vi "DFD FXP NStage MRate Code Generator.vi"(5 "open project? (F)":bool, 6 "confirm? (T)":bool=TRUE, 7 "# channels":i32=1, 8 "error in (no error)":errorcluster, 9 "filter name":string, 10 "destination folder":path, 11 "multirate filters":T1[](array[typedef]) {"mMRate_SumWl" min=1 max=32 step=1; "mMRate_InputIwl" min=1 max=32 step=1; "mMRate_GainWl" min=1 max=32 step=1; "mMRate_OutputWl" min=1 max=32 step=1; "mMRate_InputWl" min=1 max=32 step=1; "mMRate_CoefWl" min=1 max=32 step=1; "mMRate_Mode" items=["Default"=-1, "No Rate Change"=0, "Interpolation"=1, "Decimation"=2, "Interpolated"=3, "Rational"=4]}) -> (0 "error out":errorcluster, 1 "sampling frequency/FPGA clock":dbl, 2 "lvproj path":path)   [LabVIEW 2017, in "NI_DigFilterLicensed.lvlib"]
doc: "Generates LabVIEW field-programmable gate array (FPGA) code from a multistage multirate filter."
uses:
  <vilib>/addons/Digital Filter Design/NI_DigFilterLicensed.lvlib
  <vilib>/addons/Digital Filter Design/_Objects.llb/DFD Multirate Filter Obj.ctl
  <vilib>/addons/Digital Filter Design/_Objects.llb/DFD Multirate Mode.ctl
  <vilib>/addons/Digital Filter Design/_Objects.llb/DFD Coef Norm Type.ctl
  <vilib>/addons/Digital Filter Design/_Objects.llb/DFD Round-off Mode.ctl
  <vilib>/addons/Digital Filter Design/_Objects.llb/DFD FXP MRate Multiply Mode.ctl
  <vilib>/addons/Digital Filter Design/nMAC.llb/Typedefs/dfd_nMAC_Parameter.ctl
  <vilib>/addons/Digital Filter Design/nMAC.llb/Typedefs/dfd_nMAC_Memory Type.ctl
  <vilib>/addons/Digital Filter Design/nMAC.llb/Typedefs/dfd_nMAC_Coef Reload API.ctl
  <vilib>/addons/Digital Filter Design/nMAC.llb/Typedefs/dfd_nMAC_Execution Mode.ctl
  <vilib>/addons/Digital Filter Design/NI_DigFilter_CodeGen.lvlib
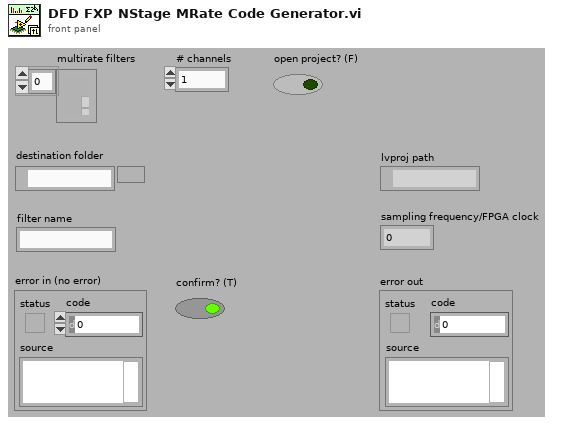
[diagram p1: front panel]
types:
  T1 = typedef "NI_DigFilterLicensed.lvlib/DFD Multirate Filter Obj.ctl" = cluster{"mMRate_Structure":enum16{"CIC", "FIR", "IIR", "Lattice"}, "mMRate_Mode":T2, "mMRate_Factor":i32, "mMRate_FIRParams":cluster{"mMRate_FIR_H":dbl[], "mMRate_FIR_IsNyquist?":bool, "mMRate_FIR_IsSymmetric?":bool}, "mMRate_CICParams":cluster{"mMRate_CIC_#Stage":i32, "mMRate_CIC_Lag":i32, "mMRate_CIC_Type":enum16{"Lowpass", "Highpass"}}, "mMRate_Order":i32, "mMRate_Version":string, "mMRate_Comments":string, "mMRate_RationalFactor":cluster{"mMRate_L":i32, "mMRate_M":i32}, "mMRate_Fs":dbl, "mMRate_Quantized?":bool, "mMRate_QFilterGain":dbl, "mMRate_CoefWl":i16, "mMRate_Scaling":cluster{"mMRate_ScaleByPowerOf2?":bool, "mMRate_ScaleType":T3}, "mMRate_InputWl":i16, "mMRate_OutputWl":i16, "mMRate_OutputMode":T4, "mMRate_MultMode":T5, "mMRate_BitPruning":bool, "mMRate_GainWl":i16, "mMRate_OutputFwl":i16, "mMRate_SumIwl":i16, "mMRate_InputIwl ":i16, "mMRate_SumWl":i16, "mMRate_CoefIwl":i16}
  T2 = typedef "NI_DigFilterLicensed.lvlib/DFD Multirate Mode.ctl" = i16
  T3 = typedef "NI_DigFilterLicensed.lvlib/DFD Coef Norm Type.ctl" = enum16{"No Norm", "Time Domain 1-Norm", "Time Domain 2-Norm", "Time Domain Inf-Norm"}
  T4 = typedef "NI_DigFilterLicensed.lvlib/DFD Round-off Mode.ctl" = enum16{"Nearest", "Truncation"}
  T5 = typedef "NI_DigFilterLicensed.lvlib/DFD FXP MRate Multiply Mode.ctl" = enum16{"Truncated", "Full"}
  T6 = typedef "dfd_nMAC_Execution Mode.ctl" = enum16{"Outside SCTL", "Inside SCTL"}
  T7 = typedef "dfd_nMAC_Parameter.ctl" = cluster{"#MACs":u32, "#level per register":u32, "#multiply pipeline stage":u32, "multiply register in":bool, "#paths":u32, "state memory":T8, "coefficient memory":T8, "coefficient reloadable":bool, "coefficient reload API":T9}
  T8 = typedef "dfd_nMAC_Memory Type.ctl" = enum16{"Automatic", "BRAM", "DRAM"}
  T9 = typedef "dfd_nMAC_Coef Reload API.ctl" = enum16{"Multiple interfaces", "Single interface"}
  T10 = typedef "dfd_nMAC_Implementation Parameter.ctl" = cluster{"common parameters":cluster{"execution mode":T6, "number of channels":u32, "reset":bool, "include overflow status":bool, "4-wire":bool}, "specific parameters":cluster{"number of MACs":u32, "multiply pipeline stages":u32, "multiply register in":bool, "#level per register":u32, "state memory":T8, "coefficient memory":T8, "number of paths":u32, "coefficient reloadable":bool, "coefficient reload API":T9, "coef map type":T11, "set vs channel map":u32[]}}
  T11 = typedef "dfd_nMAC_Coef Map Type.ctl" = enum16{"No Map", "Set Map", "Channel Map"}
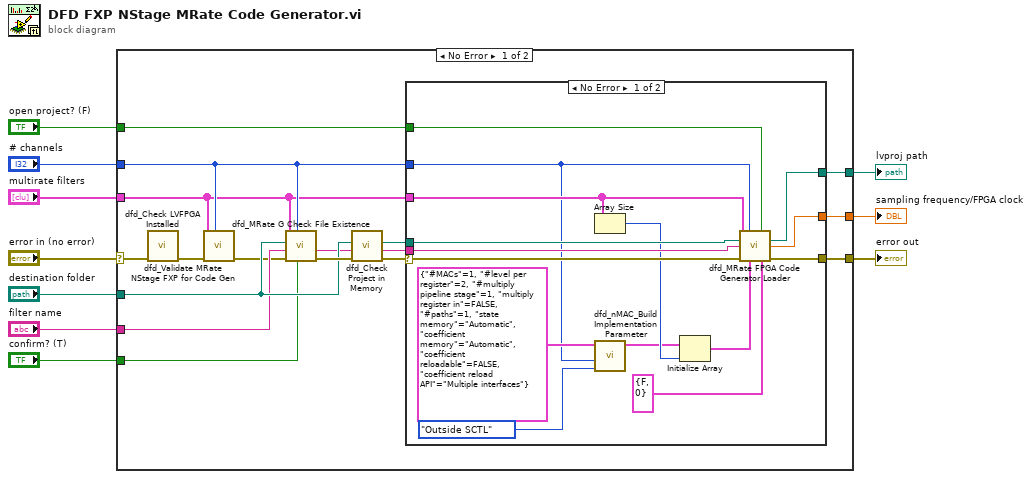
[diagram p0: block diagram]
diagram:
  n1 = case shown="No Error" "error in (no error)" {
    selector: "error in (no error)" -> [w11 w44]
    tunnel: [w27 _] -> w10
    tunnel: [w26 w44] -> w9
    tunnel: [w23 _] -> w8
    tunnel: "destination folder" -> [w21 _]
    tunnel: "confirm? (T)" -> [w20 _]
    tunnel: "open project? (F)" -> [w19 _]
    tunnel: "# channels" -> [w18 _]
    tunnel: "filter name" -> [w17 _]
    tunnel: "multirate filters" -> [w12 _]
    frame No Error {
      n2 = call <vilib>:"dfd_Check LVFPGA Installed.vi"("error in (no error)"=w11) -> ("error out"=w16:errorcluster)  [unwired: 10 out]
      n3 = call <vilib>:"dfd_Validate MRate NStage FXP for Code Gen.vi"("totalChan"=w18, "error in"=w16, "multirate filters"=w12) -> ("error out"=w15:errorcluster)  [unwired: 8 out]
      n4 = call <vilib>:"dfd_MRate G Check File Existence.vi"("confirm?"=w20, "# channels"=w18, "error in (no error)"=w15, "filter name"=w17, "dest path"=w21, "multirate filters"=w12) -> ("error out"=w22:errorcluster, "filter name out"=w13:string)  [unwired: 4 out]
      n5 = call <vilib>:"dfd_Check Project in Memory.vi"("error in (no error)"=w22, "filter name"=w13, "dest path"=w21) -> ("error out"=w14:errorcluster, "filter name out"=w24:string, "dup dest path"=w25:path)  [unwired: 6 out]
      n6 = case shown="No Error" w14 {
        selector: w14 -> [w39 w43]
        tunnel: w12 -> [w34 _]
        tunnel: w25 -> [w40 _]
        tunnel: w24 -> [w41 _]
        tunnel: w18 -> [w30 _]
        tunnel: [w38 _] -> w27
        tunnel: [w42 w43] -> w26
        tunnel: [w37 _] -> w23
        tunnel: w19 -> [w36 _]
        frame No Error {
          n7 = Array Size(array=w34) -> (size(s)=w33:i32)
          n8 = call <vilib>:"dfd_nMAC_Build Implementation Parameter.vi"("execution mode"=dfd_nMAC_Execution_Mode."Outside SCTL", "# channels"=w30, "nMAC Parameters"=T7 {"#MACs"=1, "#level per register"=2, "#multiply pipeline stage"=1, "multiply register in"=FALSE, "#paths"=1, "state memory"=enum."Automatic", "coefficient memory"=enum."Automatic", "coefficient reloadable"=FALSE, "coefficient reload API"=enum."Multiple interfaces"}) -> ("implementation para in"=w28:T10)  [unwired: 8 in]
          n9 = Initialize Array(w28, w33) -> (w32:T10[])
          n10 = call <vilib>:"dfd_MRate FPGA Code Generator Loader.vi"("multirate filters"=w34, "totalChan"=w30, "open project? (F)"=w36, "destination path"=w40, "filter name"=w41, "error in (no error)"=w39, "nStage nMAC Parameters"=w32, "CIC Paramters"=cluster{"pipeline?":bool, "output phase":i32} {"pipeline?"=FALSE, "output phase"=0}) -> ("lvproj path"=w37:path, "sampling rate/FPGA clock"=w38:dbl, "error out"=w42:errorcluster)  [unwired: 5 in]
        }
        frame Error {
        }
      }
    }
    frame Error {
    }
  }
  "error out" <- w9
  "sampling frequency/FPGA clock" <- w10
  "lvproj path" <- w8
